vi "Position to Grid Index.vi"(2 "Grid Settings":T1={"X cells"=40, "Y cells"=40, "X size (m)"=0.1, "Y size (m)"=0.1}, 3 "Global Position":cluster{"Robot X (m)":dbl, "Robot Y (m)":dbl}) -> (0 "In Range?":cluster{"X cells":bool, "Y cells":bool}, 1 "Grid Index":cluster{"Sensor X":i32, "Sensor Y":i32})   [LabVIEW 2012]
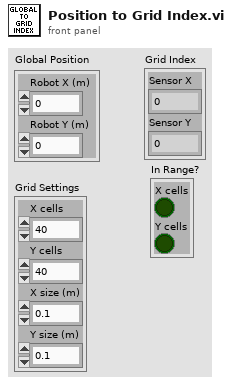
[diagram p1: front panel]
types:
  T1 = cluster{"X cells":i32, "Y cells":i32, "X size (m)":dbl, "Y size (m)":dbl}
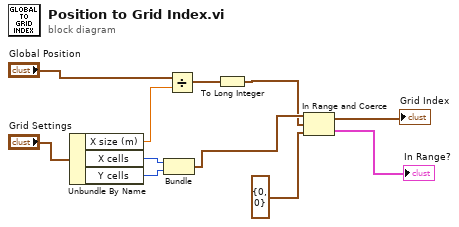
[diagram p0: block diagram]
diagram:
  n1 = Unbundle By Name("Grid Settings") -> ("X size (m)"=w8:dbl, "X cells"=w7:i32, "Y cells"=w6:i32)
  n2 = Bundle("X cells"=w7, "Y cells"=w6) -> (w5:cluster{"X cells":i32, "Y cells":i32})  [unwired: 1 in]
  n3 = Divide(x="Global Position", y=w8) -> (x/y=w11:cluster{"Robot X (m)":dbl, "Robot Y (m)":dbl})
  n4 = To Long Integer(number=w11) -> (32bit integer=w3:cluster{"Robot X (m)":i32, "Robot Y (m)":i32})
  n5 = In Range and Coerce(upper limit=w5, x=w3, lower limit=cluster{"X cells":i32, "Y cells":i32} {"X cells"=0, "Y cells"=0}) -> (coerced(x)=→"Grid Index":cluster{"X cells":i32, "Y cells":i32}, In Range?=→"In Range?":cluster{"X cells":bool, "Y cells":bool})
